vi "DAE Spring Pendulum Simulation.vi"() -> ()   [LabVIEW 2023]
doc: "This example demonstrates how to use the <B>DAE Radau 5th Order VI</B> to simulate the movement of a spring pendulum, which is modeled by a differential algebraic equation. In this example, a VI implements the model, and a strictly typed reference of that VI is passed to the solver VI."
uses:
  <vilib>/gmath/dae.llb/Radau5_Parameters.ctl
  <vilib>/Analysis/1siggen.llb/Ramp Pattern by Samples.vi
  <vilib>/gmath/dae.llb/DAE Radau 5th Order (VIRef).vi
  <vilib>/gmath/NI_DAE.lvlib
  <vilib>/gmath/NI_Gmath.lvlib
  <vilib>/Analysis/NI_AALBase.lvlib
panel:
  in  "Initial Position":dbl(slide)=0.8016949152542373 min=0.4 max=1.0 step=0.01 scale=0.4..1.0 scale format="%#_2g"
  out "pendulum":picture
  out "Spring Pendulum Simulation":picture
  # "Overview: This example demonstrates how to use the DAE Radau 5th Order VI to simulate the movement of a spring pendulum, which is modeled by a differential algebraic equation.\nRequirements: LabVIEW Full Development System\nInstructions: \n1. Run the VI. \n2. Change the Initial Position and run the VI again to see how the spring pendulum swings with different initial positions."
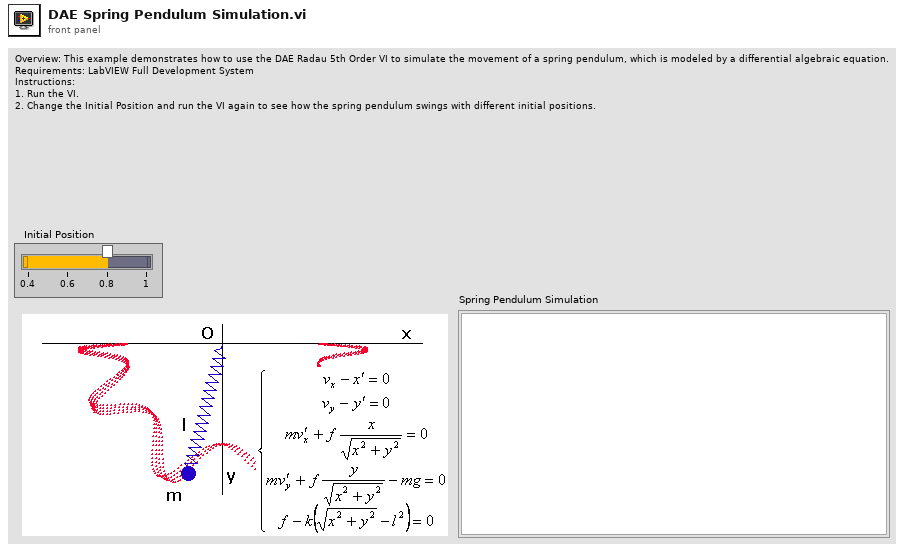
[diagram p1: front panel]
types:
  T1 = typedef "NI_DAE.lvlib/Radau5_Parameters.ctl" = cluster{"initial time":dbl, "final time":dbl, "Absolute Tolerance":dbl[], "Relative Tolerance":dbl[], "minimum time step":dbl, "maximum time step":dbl, "initial time step":dbl}
  T2 = cluster{"Width":u16, "Style":enum32{"Solid", "Dash", "Dot", "DashDot", "DashDotDot"}}
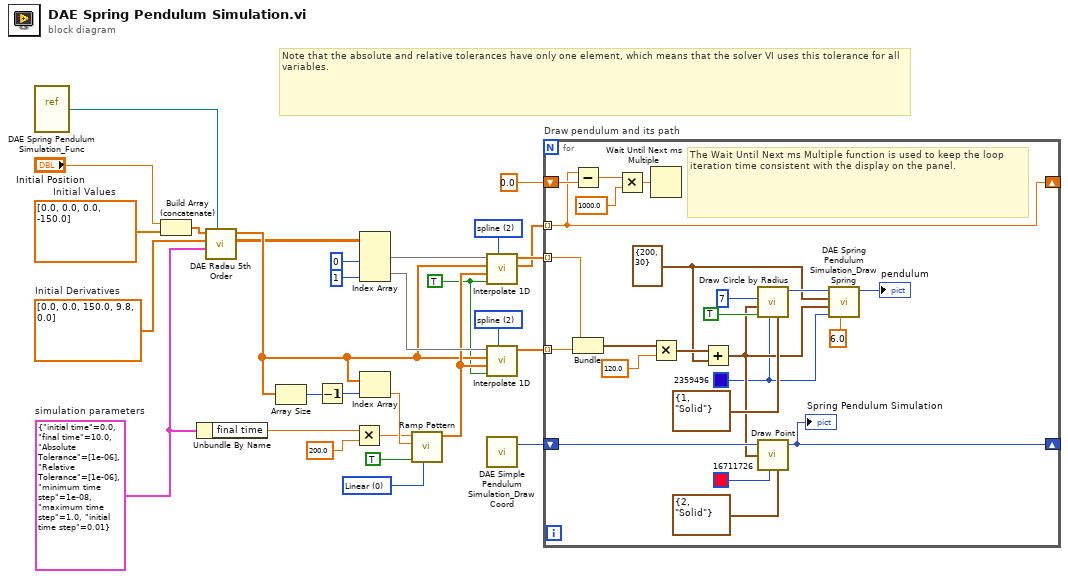
[diagram p0: block diagram]
diagram:
  w7 = T1 {"initial time"=0.0, "final time"=10.0, "Absolute Tolerance"=[1e-06], "Relative Tolerance"=[1e-06], "minimum time step"=1e-08, "maximum time step"=1.0, "initial time step"=0.01}  # simulation parameters
  w5 = TRUE ("X is monotonic")
  w28 = 2 items=["nearest", "linear", "spline", "cubic Hermite", "Lagrange"] ("method")
  w22 = 2 items=["nearest", "linear", "spline", "cubic Hermite", "Lagrange"] ("method")
  w16 = u16 0 items=["Linear", "Logarithmic"] ("type")
  w2 = dbl[] [0.0, 0.0, 0.0, -150.0]  # Initial Values
  w29 = dbl[] [0.0, 0.0, 150.0, 9.8, 0.0]  # Initial Derivatives
  # "Note that the absolute and relative tolerances have only one element, which means that the solver VI uses this tolerance for all variables."
  n1 = vi-ref "DAE Spring Pendulum Simulation_Func.vi"() -> (w4:refnum<vi>)
  n2 = Build Array (concatenate)("Initial Position", w2) -> (w1:dbl[])
  n3 = Unbundle By Name(w7) -> ("final time"=w6:dbl)
  n4 = call-poly <vilib>:"DAE Radau 5th Order.vi"("DAE F(X,X',t)"=w4, "simulation parameters"=w7, "Initial Derivatives"=w29, "Initial Values"=w1) -> ("X Values"=w10:dbl[][], "Times"=w11:dbl[])  [unwired: 4 in, 2 out]
  n5 = Array Size(array=w11) -> (size(s)=w24:i32)
  n6 = Decrement(x=w24) -> (x-1=w23:i32)
  n7 = Multiply(x=w6, y=200.0 ("samples")) -> (x*y=w8:dbl)
  n8 = Index Array(array=w10, index (col) #1=0 ("disabled index (col)"), index (col) #2=1 ("index (col)")) -> (element #1=w18:dbl[], element #2=w27:dbl[])  [unwired: 2 in]
  n9 = Index Array(array=w11, index=w23) -> (element=w25:dbl)
  n10 = call-poly <vilib>:"Ramp Pattern.vi"("type"=w16, "exclude end?"=TRUE, "end"=w25, "samples"=w8) -> ("Ramp Pattern"=w20:dbl[])  [unwired: 6 in, 1 out]
  n11 = call <vilib>:"Interpolate 1D.vi"("method"=w22, "X is monotonic"=w5, "xi"=w20, "X"=w11, "Y"=w18) -> ("xi used"=w17:dbl[], "yi"=w19:dbl[])  [unwired: 1 in, 4 out]
  n12 = call <vilib>:"Interpolate 1D.vi"("method"=w28, "X is monotonic"=w5, "xi"=w20, "X"=w11, "Y"=w27) -> ("yi"=w21:dbl[])  [unwired: 1 in, 5 out]
  n13 = call "DAE Simple Pendulum Simulation_Draw Coord.vi"() -> ("picture out"=w13:picture)  [unwired: 3 in]
  n14 = for "Draw pendulum and its path" {
    tunnel: w17 -> [w37] mode=indexing
    tunnel: w19 -> [w52] mode=indexing
    tunnel: w21 -> [w38] mode=indexing
    shift-right: [w43] -> _
    shift-left: w13 -> [w44]
    shift-right: [w37] -> _
    shift-left: 0.0 -> [w40]
    w33 = u32 2359496 ("color(black)")
    w35 = cluster{i16, i16} {200, 30} ("y")
    # "The Wait Until Next ms Multiple function is used to keep the loop iteration time consistent with the display on the panel."
    n15 = Subtract(x=w37, y=w40) -> (x-y=w39:dbl)
    n16 = Bundle("Numeric"=w52, "Numeric"=w38) -> (w51:cluster{"Numeric":dbl, "Numeric":dbl})  [unwired: 1 out]
    n17 = Multiply(x=w39, y=1000.0) -> (x*y=w36:dbl)
    n18 = Wait Until Next ms Multiple(millisecond multiple=w36) -> ()  [unwired: 1 out]
    n19 = Multiply(x=w51, y=120.0) -> (x*y=w49:cluster{"Numeric":dbl, "Numeric":dbl})
    n20 = Add(x=w49, y=w35) -> (x+y=w34:cluster{dbl, dbl})
    n21 = call <vilib>:"Draw Circle by Radius.vi"("pen"=T2 {"Width"=1, "Style"=enum."Solid"}, "color(black)"=w33, "fill?(F)"=TRUE, "pixel center"=w34, "radius"=i16 7) -> ("new picture"=w46:picture)  [unwired: 3 in, 3 out]
    n22 = call <vilib>:"Draw Point.vi"("picture"=w44, "point(x,y)"=w34, "color(black)"=u32 16711726, "pen"=T2 {"Width"=2, "Style"=enum."Solid"}) -> ("new picture"=w43:picture)  [unwired: 5 out]
    "Spring Pendulum Simulation" <- w43
    n23 = call "DAE Spring Pendulum Simulation_Draw Spring.vi"("width"=6.0, "color(blue)"=w33, "End point"=w34, "Start point"=w35, "picture in"=w46) -> ("picture out"=→"pendulum":picture)  [unwired: 6 in]
  }
